vi "SSH_Write.vi"(8 "error in (no error)":errorcluster, 10 "Text to write":string, 11 "Python":T1) -> (0 "error out":errorcluster, 3 "Python":T1)   [LabVIEW 2022 SP3]
uses:
  PythonCtrl.ctl
  Processors.ctl
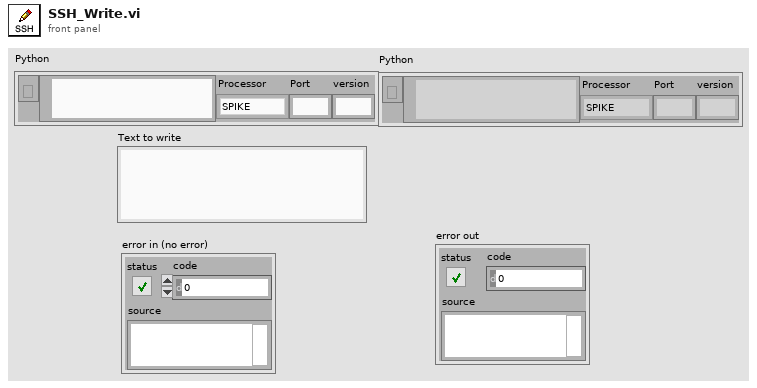
[diagram p1: front panel]
types:
  T1 = typedef "PythonCtrl.ctl" = cluster{"session":refnum<k35>, "PyPath":path, "Processor":T2, "Port":string, "version":string}
  T2 = typedef "Processors.ctl" = enum16{"SPIKE", "Pi", "Pi_ssh", "OpenMV", "Dunio"}
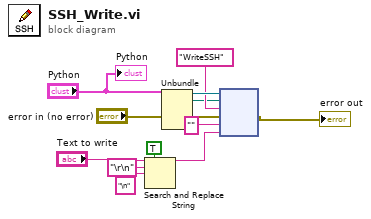
[diagram p0: block diagram]
diagram:
  n1 = Search and Replace String(replace all?=TRUE ("replace all? (F)"), input string="Text to write", search string="\r\n", replace string="\n" ("search string")) -> (result string=w11:string)  [unwired: 4 in, 3 out]
  n2 = Unbundle("Python") -> ("session"=w12:refnum<k35>, "PyPath"=w2:path)  [unwired: 3 out]
  n3 = node(w12, w2, "WriteSSH" ("function name"), "error in (no error)", "" ("function name"), w11) -> (→"error out":errorcluster)  [unwired: 2 in, 3 out]
  "Python" <- "Python"
